vi "telnetTest.vi"() -> ()   [LabVIEW 2011, in "run.lvlib"]
uses:
  run.lvlib
  HWController/Network Controllers/Telnet/Telnet.lvclass
  <vilib>/addons/internet/NI_InternetTK_Core_VIs.lvlib
panel:
  in  "Read?":bool=TRUE
  in  "stop":bool
  out "reply":string
  in  "command":string="pwd"
  out "Array":string[](array[string])
  out "output":string
  out "error out":errorcluster
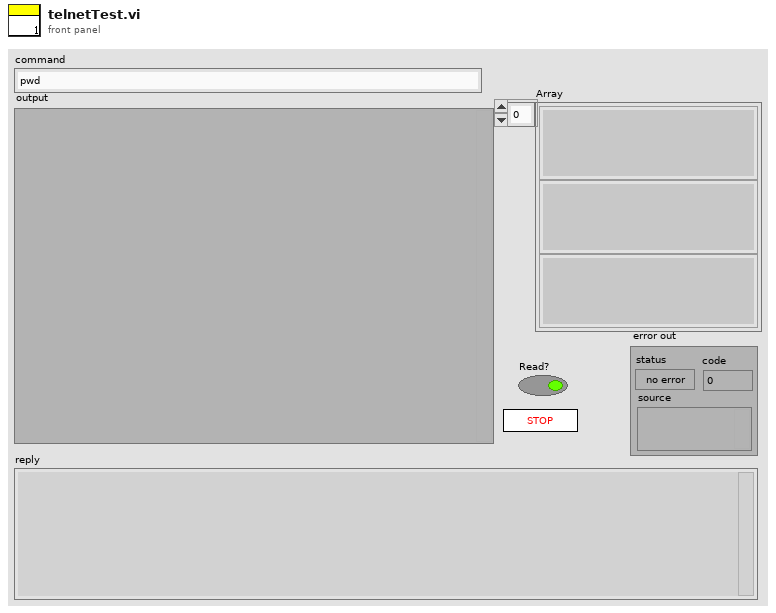
[diagram p1: front panel]
types:
  T1 = typedef "Telnet Session.ctl" = refnum<k1>
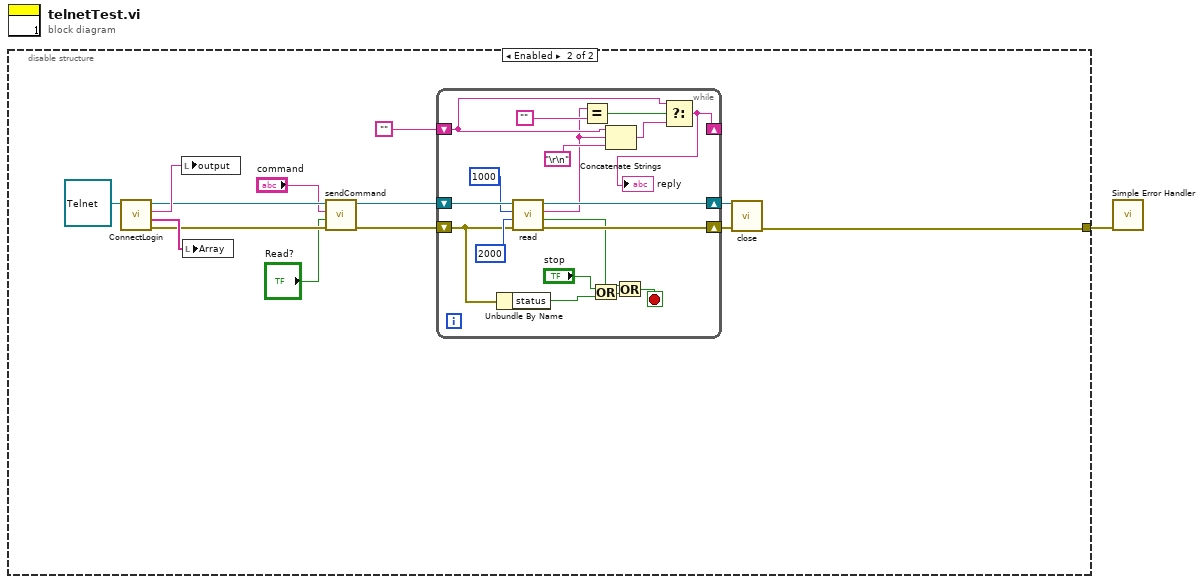
[diagram p0: block diagram]
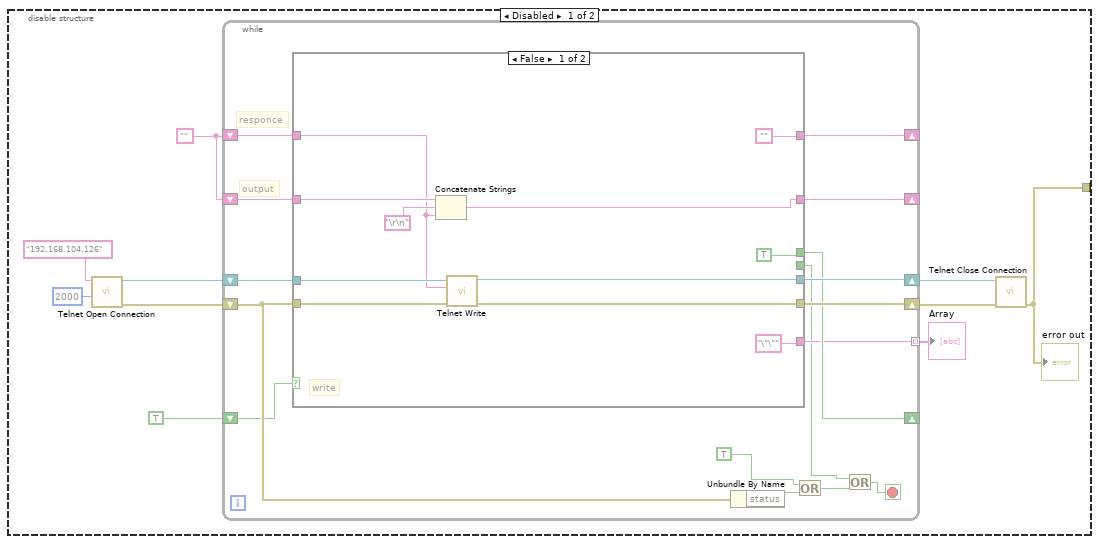
[diagram p2: hidden frame]
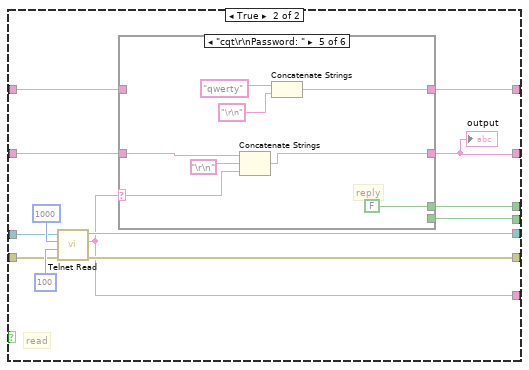
[diagram p3: hidden frame]
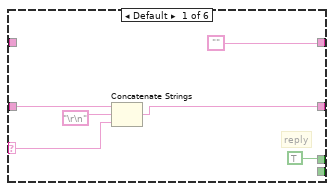
[diagram p4: hidden frame]
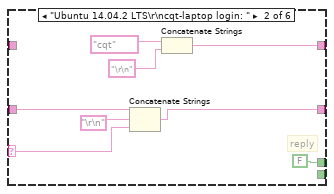
[diagram p5: hidden frame]
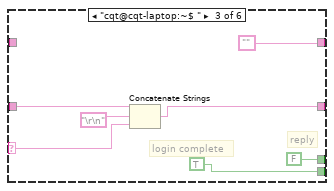
[diagram p6: hidden frame]
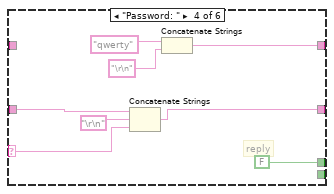
[diagram p7: hidden frame]
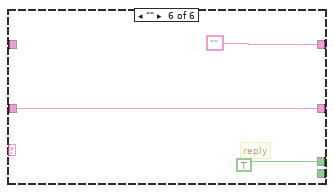
[diagram p8: hidden frame]
diagram:
  n1 = disable-structure shown="Enabled" {
    disable-tunnel: [w9 w104] -> w1
    frame Disabled {
      w5 = ""
      n2 = call <vilib>:"Telnet Open Connection.vi"("timeout ms (60000)"=2000, "address"="192.168.104.126" ("Address")) -> ("error out"=w3:errorcluster, "telnet connection"=w4:T1)  [unwired: 8 in]
      n3 = while {
        shift-right: [w26] -> w8
        shift-left: w4 -> [w27]
        shift-right: [w25] -> w7
        shift-left: w3 -> [w23]
        shift-right: [w21] -> _
        shift-left: w5 -> [w22]
        shift-right: [w19] -> _
        shift-left: TRUE -> [w20]
        shift-right: [w18] -> _
        shift-left: w5 -> [w17]
        tunnel: [w16] -> w2 mode=indexing
        stop <- w13 stop-if-true
        # "output"
        # "responce"
        n4 = case shown="False" w20 {
          tunnel: w27 -> [w37 w49]
          tunnel: [w34 w48] -> w26
          tunnel: [w35 w47] -> w25
          tunnel: w23 -> [w36 w46]
          tunnel: w22 -> [w32 w45]
          tunnel: [w31 w44] -> w21
          tunnel: [TRUE w43] -> w19
          tunnel: ["" w42] -> w18
          tunnel: w17 -> [w30 w41]
          tunnel: ["\"\"" w40] -> w16
          tunnel: [_ w39] -> w14
          frame False {
            # "write"
            n5 = Concatenate Strings(w32, "\r\n", w30) -> (w31:string)
            n6 = call <vilib>:"Telnet Write.vi"("error in (no error)"=w36, "data in"=w30, "telnet connection"=w37) -> ("error out"=w35:errorcluster, "telnet connection out"=w34:T1)  [unwired: 4 in, 1 out]
          }
          frame True {
            # "read"
            n7 = call <vilib>:"Telnet Read.vi"("error in (no error)"=w46, "timeout ms (25000)"=100, "bytes to read"=1000, "telnet connection"=w49) -> ("error out"=w47:errorcluster, "data out"=w40:string, "telnet connection out"=w48:T1)  [unwired: 3 out]
            n8 = case shown="\"cqt\\r\\nPassword: \"" w40 {
              selector: w40 -> [w54 w61 w68 w76 w84 _]
              tunnel: w45 -> [w56 w63 w70 w78 w86 w91]
              tunnel: [w55 w62 w69 w77 w85 w91] -> w44
              tunnel: [TRUE FALSE FALSE FALSE FALSE TRUE] -> w43
              tunnel: ["" w58 "" w73 w81 ""] -> w42
              tunnel: w41 -> [_ _ _ _ _ _]
              tunnel: [_ _ TRUE _ _ _] -> w39
              frame Default {
                # "reply"
                n9 = Concatenate Strings(w56, "\r\n", w54) -> (w55:string)
              }
              frame "Ubuntu 14.04.2 LTS\r\ncqt-laptop login: " {
                # "reply"
                n10 = Concatenate Strings(w63, "\r\n", w61) -> (w62:string)
                n11 = Concatenate Strings("cqt", "\r\n") -> (w58:string)
              }
              frame "cqt@cqt-laptop:~$ " {
                # "login complete"
                # "reply"
                n12 = Concatenate Strings(w70, "\r\n", w68) -> (w69:string)
              }
              frame "Password: " {
                # "reply"
                n13 = Concatenate Strings(w78, "\r\n", w76) -> (w77:string)
                n14 = Concatenate Strings("qwerty", "\r\n") -> (w73:string)
              }
              frame "cqt\r\nPassword: " {
                # "reply"
                n15 = Concatenate Strings(w86, "\r\n", w84) -> (w85:string)
                n16 = Concatenate Strings("qwerty", "\r\n") -> (w81:string)
              }
              frame "" {
                # "reply"
              }
            }
            "output" <- w44
          }
        }
        n17 = Unbundle By Name(w23) -> ("status"=w24:bool)
        n18 = Or(x=TRUE, y=w24) -> (x .or. y?=w15:bool)
        n19 = Or(x=w14, y=w15) -> (x .or. y?=w13:bool)
      }
      "Array" <- w2
      n20 = call <vilib>:"Telnet Close Connection.vi"("error in (no error)"=w7, "telnet connection"=w8) -> ("error out"=w9:errorcluster)  [unwired: 8 in, 1 out]
      "error out" <- w9
    }
    frame Enabled {
      n21 = call "ConnectLogin.vi"("Telnet in"=refnum<class "Telnet.lvclass"> refnum) -> ("error out"=w99:errorcluster, "Array"=w101:string[], "output"=w102:string, "Telnet out"=w100:refnum<class "Telnet.lvclass">)  [unwired: 7 in]
      n22 = local write "output"(w102) -> ()
      n23 = local write "Array"(w101) -> ()
      n24 = call "sendCommand.vi"("error in (no error)"=w99, "Read?"="Read?", "command"="command", "Telnet in"=w100) -> ("error out"=w96:errorcluster, "Telnet out"=w97:refnum<class "Telnet.lvclass">)  [unwired: 5 in, 1 out]
      n25 = while {
        shift-right: [w118] -> w94
        shift-left: w97 -> [w122]
        shift-right: [w119] -> w95
        shift-left: w96 -> [w117]
        shift-right: [w110] -> _
        shift-left: "" -> [w109]
        stop <- w105 stop-if-true
        n26 = Unbundle By Name(w117) -> ("status"=w116:bool)
        n27 = call "read.vi"("error in (no error)"=w117, "timeout (s)"=2000, "buffer size"=1000, "Telnet in"=w122) -> ("error out"=w119:errorcluster, "finished"=w106:bool, "read"=w108:string, "Telnet out"=w118:refnum<class "Telnet.lvclass">)  [unwired: 4 in]
        n28 = Equal?(x=w108, y="") -> (x = y?=w111:bool)
        n29 = Or(x="stop", y=w116) -> (x .or. y?=w107:bool)
        n30 = Concatenate Strings(w109, w108, "\r\n") -> (w113:string)
        n31 = Or(x=w106, y=w107) -> (x .or. y?=w105:bool)
        n32 = Select(t=w109, s=w111, f=w113) -> (s? t:f=w110:string)
        "reply" <- w110
      }
      n33 = call "close.vi"("error in (no error)"=w95, "Telnet in"=w94) -> ("error out"=w104:errorcluster)  [unwired: 8 in, 1 out]
    }
  }
  n34 = call <vilib>:"Simple Error Handler.vi"("error in (no error)"=w1) -> ()  [unwired: 4 in, 5 out]
